vi "SEP.vi"(0 "System no.":i32=1 min=1 max=4 step=1, 2 "Axis to set":string[](array[string]), 3 "Parameter value":dbl[](array[numeric]) format="%.6f", 4 "No.of digits":i16=4, 5 "error in":errorcluster, 6 "Parameter number":i32[](array[numeric]), 7 "Parameter number (hex)":u32[](array[numeric]) format="%.0x", 8 "Parameter string":string[](array[string]), 9 "Parameter no. format \n(Decimal: FALSE)":bool, 10 "Parameter format \n(Num.: FALSE)":bool, 11 "Password":string="100") -> (14 "Controller error":bool, 19 "error out":errorcluster)   [LabVIEW 2020]
doc: "If Password is correct, this VI sets parameters for commanded axes to EPROM, waits 100 ms and queries ERR?. For axis-related parameters, Axis to set is the axis name; for piezo- or sensor-related parameters, the channel number; otherwise a parameter-related code. If parameter number is in decimal format, use Parameter number input, for hexadecimal parameter numbers use Parameter number (hex.) input and switch Parameter no. format to TRUE. For numeric parameter values use Parameter value input, for parameter strings use Parameter string input and switch Parameter format to TRUE. Do not mix decimal and hex. parameter numbers or numeric and string parameter values in one call. Parameter numbers which can be set depend on current CCL level. Use HPA?.vi to get valid parameter numbers or see GCS DLL manual for available parameter numbers and values. No. of digits is the number of digits after the decimal point in the numeric parameter value(s) that will be sent. Hidden error is TRUE if selected system reports error code which is not 0. \n\nNote: This command sets the same parameters as SPA, but SPA writes them only to volatile memory, while SEP only writes to non-volatile memory. After parameters were set with SEP, use RPA to activate them (write them to volatile memory), or they become active after next power up.\n\nC-413: Parameter no. format is TRUE (hex.). Required command level depends on parameter (CCL.vi). Do not set more than 4 parameter no. at once.\n\nC-867, C-877, C-891, E-135, E-871, E-872, E-873, E-874, Mercury_GCS: Parameter no. format is TRUE (hex.). You can write only one single parameter per SEP command. See User manual for more information.\n\nC-884: Parameter no. format is TRUE (hex.). You can write up to four single parameters per SEP command. See User manual for more information.\n\nE-517, E-518: Parameter no. format is TRUE (hex.). Requires command level 1 (CCL.vi) for parameter 0X02000000 (used to enable/disable axes which is only required if the hardware configuration is changed), 0x04000E00 and 0x04000E01 (used to configure unit and format of the LCD display on the E-517 front panel).\n\nE-709: Parameter no. format is TRUE (hex.). You can write only one single parameter per SEP command. Required command level depends on parameter (CCL.vi)\n\nE-710: Parameter no. format is TRUE (hex.). Command is available in command level 1 only (see CCL.vi, CCL?.vi). Command writes parameters to Eprom and RAM\n\nE-755, E-761: Parameter no. format is TRUE (hex.)\n\nE-712, E-725, E-727, E-753, E-754: Parameter no. format is TRUE (hex.). Requires command level 1 (CCL.vi). Do not set more than 10 parameters at once. \n\nE-861: Parameter no. format is TRUE (hex.). You can write only one single parameter per SEP command. The GEMAC parameters (ID 0x7000010 to ID 0x700001F) can not be changed with SEP. Use SPA and WPA instead to save their values to non-volatile memory. See \"GEMAC Parameter Adjustment\" in the E-861 User manual for more information.\n\nE-870: Parameter no. format is TRUE (hex.). You can write only one single parameter per SEP command."
panel:
  # "If password is correct, this vi writes parameters for commanded axes to EPROM, waits 100 ms and queries ERR?. If parameter \nno. is in decimal format, use \"Parameter no.\" input, for hexadecimal parameter numbers use \"Parameter no. (hex)\" input and \nswitch \"Parameter no. format\" to TRUE. For numeric parameter values use \"Parameter value\" input, for parameter strings use\n\"Parameter string\" input and switch \"Parameter format\" to TRUE. Do not mix decimal and hex. parameter numbers or numeric \nand string parameter values in one call. See system manual for available parameter numbers and values."
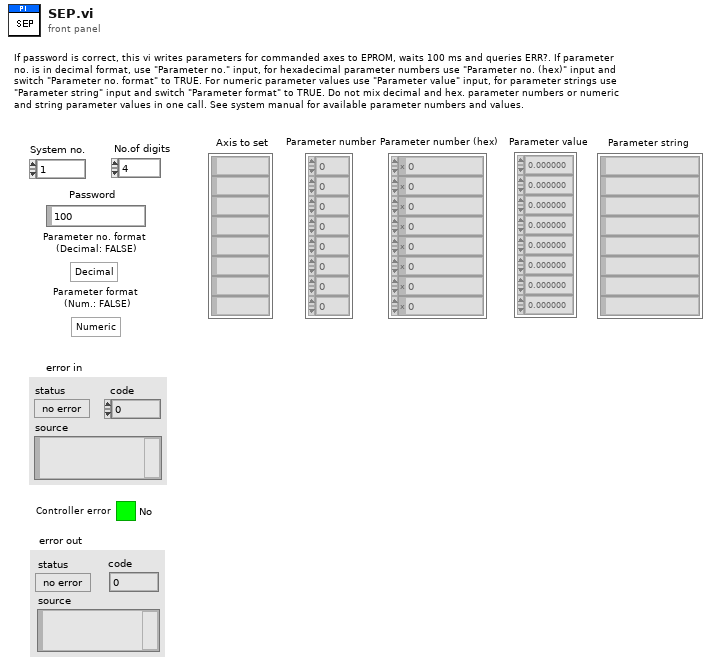
[diagram p1: front panel]
types:
  T1 = enum16{"Disable error check", "Force error check", "Use global settings"}
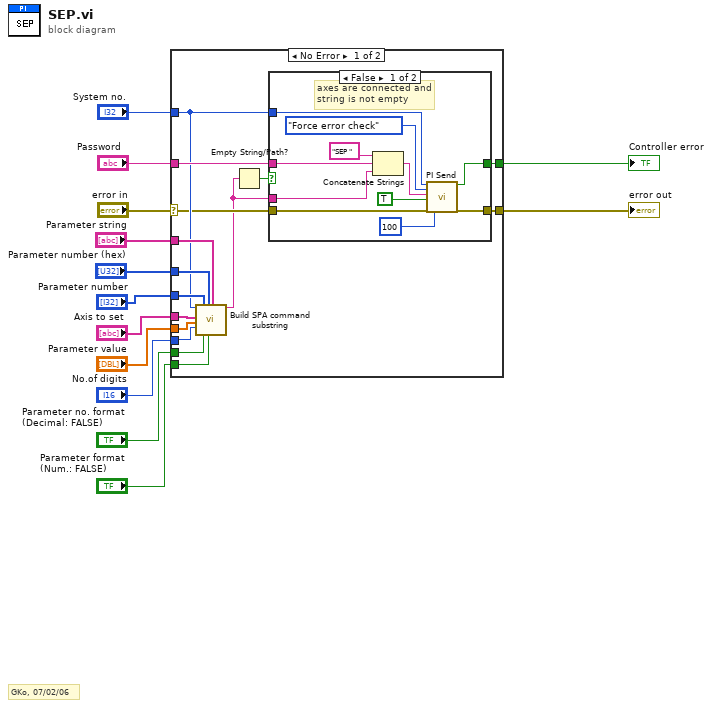
[diagram p0: block diagram]
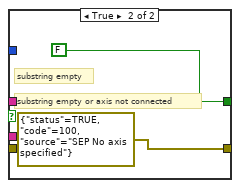
[diagram p2: hidden frame]
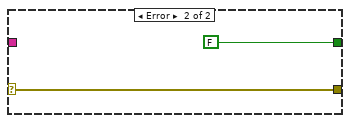
[diagram p3: hidden frame]
diagram:
  # "GKo, 07/02/06"
  n1 = case shown="No Error" "error in" {
    selector: "error in" -> [w17 w43]
    tunnel: [w28 w43] -> w13
    tunnel: "Parameter value" -> [w27 _]
    tunnel: "No.of digits" -> [w26 _]
    tunnel: "System no." -> [w20 _]
    tunnel: "Axis to set" -> [w25 _]
    tunnel: "Parameter number" -> [w24 _]
    tunnel: "Parameter string" -> [w23 _]
    tunnel: "Parameter number (hex)" -> [w22 _]
    tunnel: "Password" -> [w21 _]
    tunnel: "Parameter no. format \n(Decimal: FALSE)" -> [w19 _]
    tunnel: "Parameter format \n(Num.: FALSE)" -> [w18 _]
    tunnel: [w16 FALSE ("Controller error")] -> w1
    frame No Error {
      n2 = call "Build SPA command substring.vi"("System no."=w20, "Axes to set"=w25, "Parameter values"=w27, "No. of digits"=w26, "Parameter number"=w24, "Parameter no. format \n(Decimal: FALSE)"=w19, "Parameter number (hex)"=w22, "Parameter format \n(Num.: FALSE)"=w18, "Parameter strings"=w23) -> ("SPA command substring"=w15:string)  [unwired: 1 in, 9 out]
      n3 = Empty String/Path?(string/path=w15) -> (empty?=w14:bool)
      n4 = case shown="False" w14 {
        tunnel: w15 -> [w34 _]
        tunnel: [w29 errorcluster {"status"=TRUE, "code"=100, "source"="SEP No axis specified"} ("error out")] -> w28
        tunnel: w17 -> [w36 _]
        tunnel: w20 -> [w35 _]
        tunnel: w21 -> [w33 _]
        tunnel: [w30 FALSE ("Controller error")] -> w16
        frame False {
          # "axes are connected and\nstring is not empty"
          n5 = Concatenate Strings("SEP ", w33, w34) -> (w37:string)
          n6 = call "PI Send.vi"("System no."=w35, "Error check settings"=T1."Force error check", "String to send"=w37, "Attach termination char.?"=TRUE ("Attach Linefeed?"), "error in"=w36, "Delay before error check (ms)"=u32 100 ("milliseconds to wait")) -> ("Controller error"=w30:bool, "error out"=w29:errorcluster)  [unwired: 12 out]
        }
        frame True {
          # "substring empty"
          # "substring empty or axis not connected"
        }
      }
    }
    frame Error {
    }
  }
  "error out" <- w13
  "Controller error" <- w1
